vi "From Variant.vi"(0 "Obj in":refnum<class "Parameters.lvclass">, 7 "Variant":variant, 9 "Prefix":string, 11 "error in (no error)":errorcluster) -> (4 "Obj out":refnum<class "Parameters.lvclass">, 15 "error out":errorcluster)   [LabVIEW 2020, in "Parameters.lvclass"]
uses:
  Parameters.lvclass
  Parameters.lvclass/Parameters.ctl
  epl-vi-lib/Koop/KObject Class/KObject.lvclass
  State/State.lvclass
  epl-vi-lib/Signal Synthesis VIs/4th Generation/Classes/Channel/Channel.lvclass
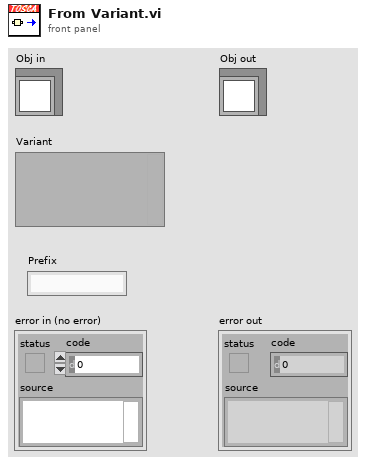
[diagram p1: front panel]
types:
  T1 = typedef "Parameters.lvclass/Serialized.ctl" = cluster{"Flowchart":refnum<class "State.lvclass">[], "First state":string, "Input Events":T2[], "Flags":T6[], "DAQ":T7, "Schedule Mode":T8, "Description":string, "MATLAB function":path, "Imaging":T9, "Connect":T11, "Adapt":T12, "Schedule":T16, "Pretrial":T21, "AI":T22, "Target state":string, "Masker":refnum<class "Channel.lvclass">, "Use masker":bool, "Link to":path}
  T2 = typedef "Tosca-Input Event.ctl" = cluster{"Name":string, "Criteria":T3[], "Operators":enum16{"AND", "OR"}[], "Accumulator":T5}
  T3 = typedef "Tosca-Input Criterion.ctl" = cluster{"DigInput":i32, "State":T4, "Time (ms)":i32, "Name":string}
  T4 = typedef "Logic State.ctl" = enum16{"Low", "High", "Rising", "Falling"}
  T5 = typedef "Tosca-Accumulator.ctl" = cluster{"active":bool, "N":i32, "T":dbl, "Imax":dbl, "latency":dbl}
  T6 = typedef "Tosca-Flag.ctl" = cluster{"Name":string, "Default":i32}
  T7 = typedef "Parameters.lvclass/DAQ.ctl" = cluster{"AO Fs (Hz)":dbl, "DO Fs (Hz)":dbl, "Poll Rate (Hz)":dbl, "Baseline (s)":dbl}
  T8 = typedef "Tosca-Schedule Mode.ctl" = enum16{"Seq", "CS+/CS-", "Adapt"}
  T9 = typedef "Tosca-Imaging.ctl" = cluster{"mode":T10, "FrameRateHz":dbl, "use AO":bool, "destination":string}
  T10 = typedef "Tosca-Imaging Mode.ctl" = enum16{"Off", "Widefield", "Two-photon"}
  T11 = typedef "Parameters.lvclass/Connect.ctl" = cluster{"Tracking":bool, "Synapse":bool, "Pupil":bool, "Loco":bool, "Retrieve":bool, "Codes":string}
  T12 = typedef "Tosca-Adapt.ctl" = cluster{"Switch after":i32, "Switch type":enum16{"Trials", "Reversals"}, "Tracks":T13[]}
  T13 = typedef "Tosca-Adaptive Track.ctl" = cluster{"state":string, "chan":string, "param":string, "Start":dbl, "Step":string, "Mode":enum16{"Add", "Multiply"}, "Pcatch":dbl, "Ndown":i32, "Nup":i32, "Nreverse":i32, "Min":dbl, "Max":dbl, "Catch":T14[], "do all catch":bool, "name":string, "Vars":T14[], "compute":T15, "of last":i32, "Step2":string, "after":i32}
  T14 = typedef "Tosca-Simple Variable.ctl" = cluster{"state":string, "chan":string, "param":string, "expr":string}
  T15 = typedef "Tosca-Adapt Threshold Metric.ctl" = enum16{"mean", "median"}
  T16 = typedef "Tosca-Schedule.ctl" = cluster{"Blocks":i32, "order":T17, "balance":bool, "Families":T18[]}
  T17 = typedef "Tosca-Sequence Order.ctl" = enum16{"Sequential", "Alternate", "Randomize", "Random group"}
  T18 = typedef "Tosca-Parameter Family.ctl" = cluster{"Name":string, "Number":i32, "Vars":T19[], "Mask":bool[][], "one each":bool}
  T19 = typedef "Tosca-Parameter Table Element.ctl" = cluster{"state":string, "chan":string, "param":string, "expr":string, "dim":T20, "value":dbl[]}
  T20 = typedef "Tosca-Parameter Dimension.ctl" = enum16{"Ind", "X", "Y"}
  T21 = typedef "Tosca-Pretrial Spec.ctl" = cluster{"Path":path, "Args":string[]}
  T22 = typedef "Tosca-AI.ctl" = cluster{"active":bool, "Fs":dbl, "AI":string[], "DI":string[]}
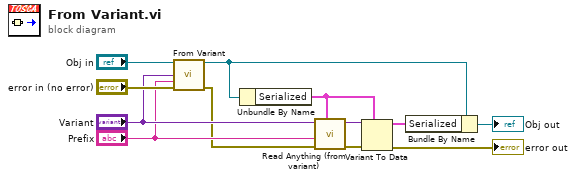
[diagram p0: block diagram]
diagram:
  n1 = call-parent "From Variant.vi"("KObject in"="Obj in", "Variant"="Variant", "Prefix"="Prefix", "error in (no error)"="error in (no error)") -> ("KObject out"=w3:refnum<class "Parameters.lvclass">, "error out"=w4:errorcluster)  [unwired: 10 in]
  n2 = Unbundle By Name(w3) -> ("Serialized"=w8:T1)
  n3 = call "Read Anything (from variant).vi"("Type of Anything"=w8, "Error In"=w4, "Prefix"="Prefix", "Variant Database"="Variant") -> ("Error Out"=w9:errorcluster, "Anything"=w10:variant)  [unwired: 5 in, 1 out]
  n4 = Variant To Data(error in=w9, type=w8, Variant=w10) -> (data=w7:T1, error out=→"error out":errorcluster)
  n5 = Bundle By Name(cluster=w3, "Serialized"=w7) -> (→"Obj out":refnum<class "Parameters.lvclass">)
